vi "Main.vi"() -> ()   [LabVIEW 2013]
uses:
  <vilib>/myRIO/Instrument Drivers/Onboard IO/AI/vis/Smart Open.vi
  <vilib>/myRIO/Instrument Drivers/Onboard IO/AI/vis/Read.vi
  <vilib>/myRIO/Common/Instrument Driver Framework/myRIO v1.0/UART/vis/myRIO v1.0 Close UART.vi
  <vilib>/myRIO/Instrument Drivers/Onboard IO/AI/vis/Open.vi
  <vilib>/myRIO/Common/Instrument Driver Framework/myRIO v1.0/AI/vis/myRIO v1.1 Open AI.vi
  <vilib>/myRIO/Common/Instrument Driver Framework/Utilities/vis/Validate Channels.vi
  <vilib>/myRIO/Common/Instrument Driver Framework/myRIO v1.0/AI/vis/myRIO v1.0 Reserve AI.vi
  <vilib>/myRIO/Common/Instrument Driver Framework/myRIO v1.0/AI/vis/myRIO v1.0 Build MUX Configuration AI.vi
  <vilib>/myRIO/Common/Instrument Driver Framework/myRIO v1.0/Resource Manager/vis/myRIO v1.0 Reserve Channel List.vi
  <vilib>/myRIO/Common/Instrument Driver Framework/myRIO v1.0/Resource Manager/vis/myRIO v1.0 Reserve Channel.vi
  <vilib>/myRIO/Common/Instrument Driver Framework/myRIO v1.0/Resource Manager/vis/myRIO v1.0 Unreserve Channel.vi
  <vilib>/myRIO/Common/Instrument Driver Framework/myRIO v1.0/Resource Manager/vis/myRIO v1.0 Build Mutex Name.vi
  <vilib>/myRIO/Common/Instrument Driver Framework/myRIO v1.0/myRIO v1.1 Open.vi
  <vilib>/myRIO/Common/Instrument Driver Framework/myRIO v1.0/AI/vis/myRIO v1.0 Get Scaling Constants AI.vi
  <vilib>/Utility/VariantDataType/GetNumericInfo.vi
  <vilib>/Utility/error.llb/Error Cluster From Error Code.vi
  <vilib>/myRIO/Common/Instrument Driver Framework/Utilities/vis/IO Manager.vi
  <vilib>/myRIO/Common/Instrument Driver Framework/Utilities/vis/Configuration Manager.vi
  <vilib>/myRIO/Common/Instrument Driver Framework/myRIO v1.0/myRIO v1.0 Close.vi
  <vilib>/myRIO/Common/Instrument Driver Framework/myRIO v1.0/AI/vis/myRIO v1.0 Read AI.vi
  <vilib>/myRIO/Common/Instrument Driver Framework/Utilities/vis/FPGA Ref Manager.vi
  <vilib>/myRIO/Common/Instrument Driver Framework/myRIO v1.0/myRIO v1.0 Reset FPGA.vi
  <vilib>/myRIO/Instrument Drivers/Utilities/Utilities.lvlib
panel:
  out "B/AI0 (Pin 3) [volts]":dbl(knob) scale=0.0..5.0
  in  "[ESC]":bool
  # "Potentiometer demo"
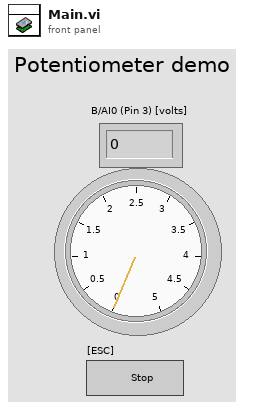
[diagram p1: front panel]
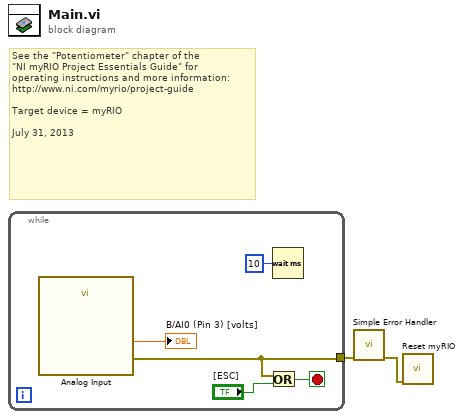
[diagram p0: block diagram]
diagram:
  # "See the \"Potentiometer\" chapter of the\n\"NI myRIO Project Essentials Guide\" for\noperating instructions and more information: \nhttp://www.ni.com/myrio/project-guide\n\nTarget device = myRIO\n\nJuly 31, 2013"
  n1 = while {
    tunnel: [w4] -> w2
    stop <- w7 stop-if-true
    n2 = call "Analog Input"() -> ("B/AI0 (Pin 3)"=→"B/AI0 (Pin 3) [volts]":dbl, "error out"=w4:errorcluster)  [unwired: 26 in]
    n3 = Or(x=w4, y="[ESC]") -> (x .or. y?=w7:bool)
    n4 = Wait (ms)(milliseconds to wait=u32 10) -> ()  [unwired: 1 out]
  }
  n5 = call <vilib>:"Simple Error Handler.vi"("error in (no error)"=w2) -> ("error out"=w1:errorcluster)  [unwired: 4 in, 4 out]
  n6 = call <vilib>:"Reset myRIO.vi"("error in (no error)"=w1) -> ()  [unwired: 10 in, 1 out]
